vi "Write Read.vi"(8 "error in (no error)":errorcluster, 10 "Frames to Write":u16[](array[numeric]), 11 "SPI Ref In":T1={"myRIO Reference"={"myRIO Model"=enum."Unknown", "myRIO Hardware Reference"={"Generic FPGA Reference"=refnum, "Allow multiple opens"=FALSE}}, "SPI Channels Enum"=enum."Not Connected", "SPI Configuration"={"Frequency [Hz]"=0.0, "Clock Phase"=enum."Leading", "Clock Polarity"=enum."Low", "Data Direction"=enum."Most significant bit first", "Frame Length"=8}} {"SPI Configuration"."Frame Length" min=1 max=16}) -> (0 "error out":errorcluster, 2 "Frames Read":u16[](array[numeric]), 3 "SPI Ref Out":T1={"myRIO Reference"={"myRIO Model"=enum."Unknown", "myRIO Hardware Reference"={"Generic FPGA Reference"=refnum, "Allow multiple opens"=FALSE}}, "SPI Channels Enum"=enum."Not Connected", "SPI Configuration"={"Frequency [Hz]"=0.0, "Clock Phase"=enum."Leading", "Clock Polarity"=enum."Low", "Data Direction"=enum."Most significant bit first", "Frame Length"=8}} {"SPI Configuration"."Frame Length" min=1 max=16})   [LabVIEW 2021, in "SPI.lvlib"]
doc: "Writes and reads data frames through a serial peripheral interface (SPI) channel at the same time. The number of data frames to write equals the number of the data frames to read."
uses:
  <vilib>/myRIO/Instrument Drivers/Onboard IO/SPI/SPI.lvlib
  <vilib>/myRIO/Instrument Drivers/Onboard IO/SPI/typedefs/SPI Reference.ctl
  <vilib>/myRIO/Common/Instrument Driver Framework/Utilities/typedefs/myRIO Generic Hardware Reference.ctl
  <vilib>/myRIO/Common/Instrument Driver Framework/Utilities/typedefs/Hardware Version Enum.ctl
  <vilib>/myRIO/Common/Instrument Driver Framework/Utilities/typedefs/myRIO v1.0 Reference.ctl
  <vilib>/myRIO/Common/Instrument Driver Framework/Utilities/typedefs/Generic FPGA Reference.ctl
  <vilib>/myRIO/Common/Instrument Driver Framework/myRIO v1.0/SPI/typedefs/SPI Channels Enum.ctl
  <vilib>/myRIO/Instrument Drivers/Onboard IO/SPI/typedefs/SPI Configuration.ctl
  <vilib>/myRIO/Common/Instrument Driver Framework/myRIO v1.0/SPI/typedefs/SPI Clock Phase.ctl
  <vilib>/myRIO/Common/Instrument Driver Framework/myRIO v1.0/SPI/typedefs/SPI Clock Polarity.ctl
  <vilib>/myRIO/Common/Instrument Driver Framework/myRIO v1.0/SPI/typedefs/SPI Data Direction.ctl
  <vilib>/myRIO/Common/Instrument Driver Framework/myRIO v1.0/SPI/typedefs/SPI Frame Length.ctl
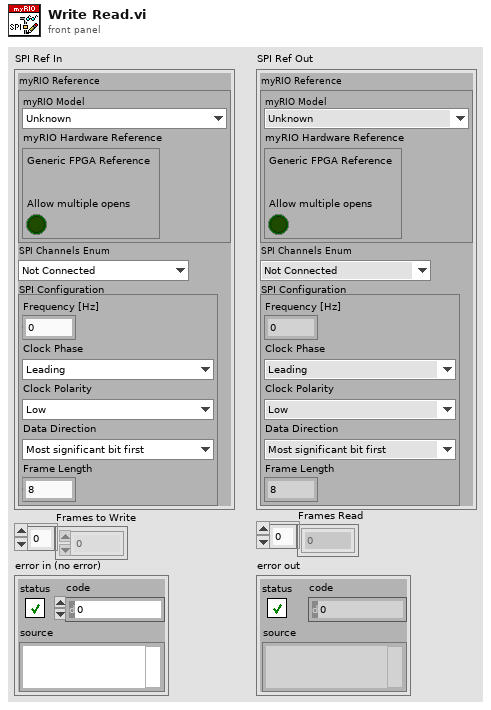
[diagram p1: front panel]
types:
  T1 = typedef "SPI.lvlib/SPI Reference.ctl" = cluster{"myRIO Reference":T2, "SPI Channels Enum":T6, "SPI Configuration":T7}
  T2 = typedef "myRIO Generic Hardware Reference.ctl" = cluster{"myRIO Model":T3, "myRIO Hardware Reference":T4}
  T3 = typedef "Hardware Version Enum.ctl" = enum16{"Unknown", "myRIO-1900", "myRIO-1950", "roboRIO", "NI ELVIS RIO CM", "ELVIS III"}
  T4 = typedef "myRIO v1.0 Reference.ctl" = cluster{"Generic FPGA Reference":T5, "Allow multiple opens":bool}
  T5 = typedef "Generic FPGA Reference.ctl" = refnum<k20>
  T6 = typedef "SPI Channels Enum.ctl" = enum16{"Not Connected", "A/SPI", "B/SPI", "SPI/SPI"}
  T7 = typedef "SPI.lvlib/SPI Configuration.ctl" = cluster{"Frequency [Hz]":dbl, "Clock Phase":T8, "Clock Polarity":T9, "Data Direction":T10, "Frame Length":T11}
  T8 = typedef "SPI Clock Phase.ctl" = enum8{"Leading", "Trailing"}
  T9 = typedef "SPI Clock Polarity.ctl" = enum8{"Low", "High"}
  T10 = typedef "SPI Data Direction.ctl" = enum8{"Most significant bit first", "Least significant bit first"}
  T11 = typedef "SPI Frame Length.ctl" = u8
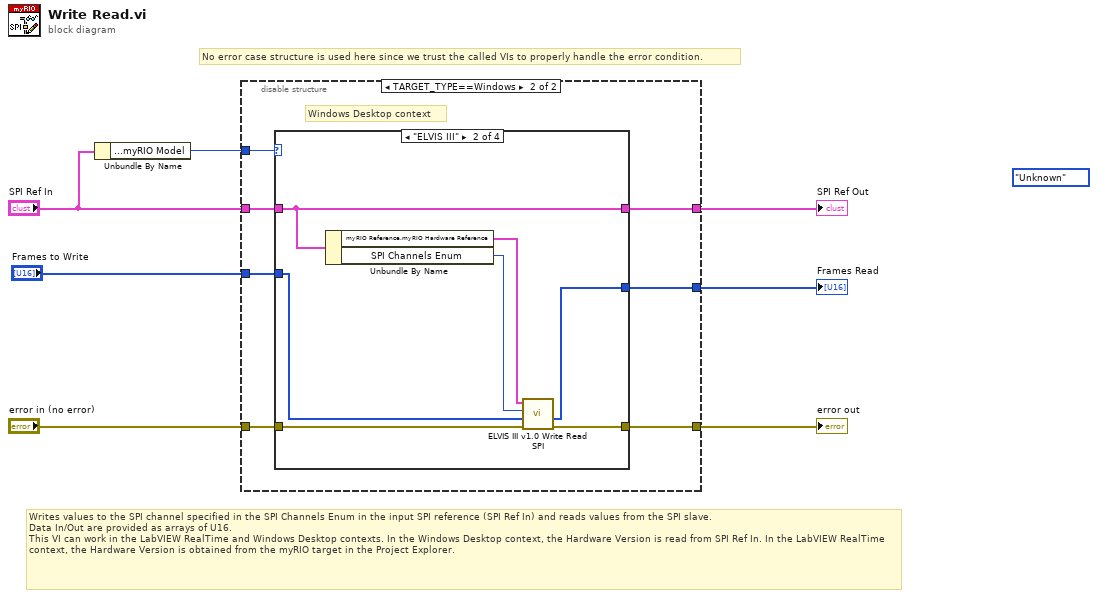
[diagram p0: block diagram]
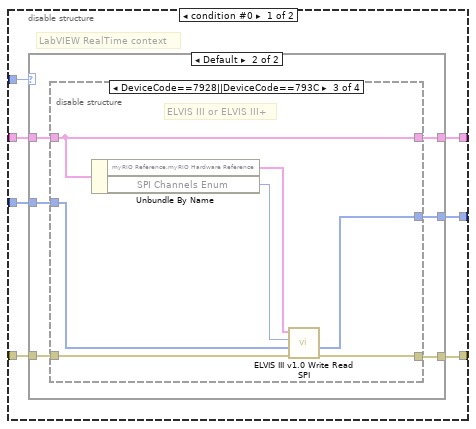
[diagram p2: hidden frame]
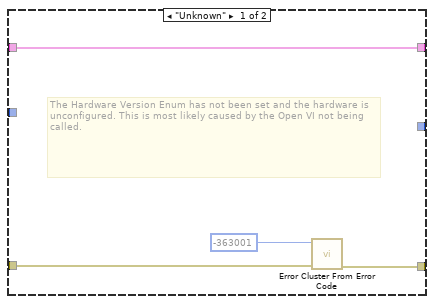
[diagram p3: hidden frame]
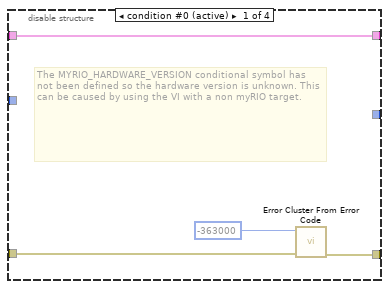
[diagram p4: hidden frame]
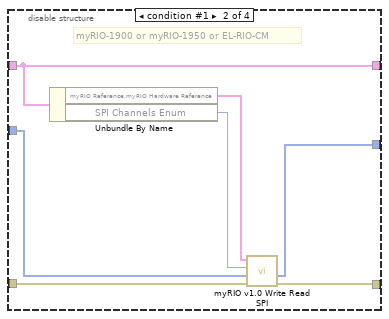
[diagram p5: hidden frame]
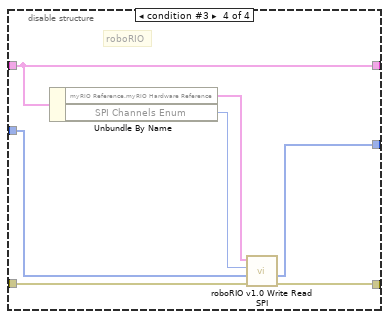
[diagram p6: hidden frame]
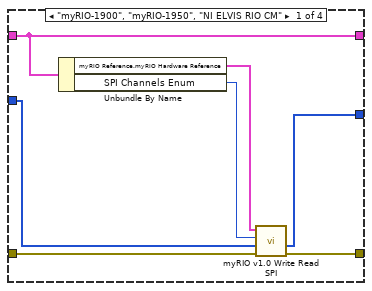
[diagram p7: hidden frame]
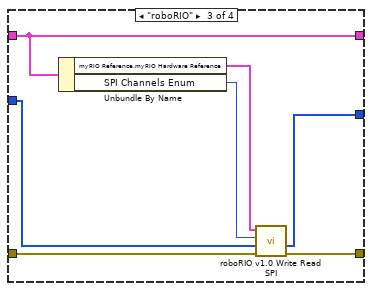
[diagram p8: hidden frame]
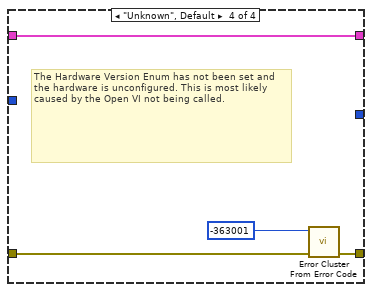
[diagram p9: hidden frame]
diagram:
  (unwired) Hardware_Version_Enum."Unknown" ("myRIO Reference.myRIO Model")
  # "No error case structure is used here since we trust the called VIs to properly handle the error condition."
  # "Writes values to the SPI channel specified in the SPI Channels Enum in the input SPI reference (SPI Ref In) and reads values from the SPI slave.\nData In/Out are provided as arrays of U16.\nThis VI can work in the LabVIEW RealTime and Windows Desktop contexts. In the Windows Desktop context, the Hardware Version is read from SPI Ref In. In the LabVIEW RealTime context, the Hardware Version is obtained from the myRIO target in the Project Explorer."
  n1 = Unbundle By Name("SPI Ref In") -> ("myRIO Reference.myRIO Model"=w1:T3)
  n2 = disable-structure shown="TARGET_TYPE==Windows" {
    disable-tunnel: [w14 w56] -> w4
    disable-tunnel: "SPI Ref In" -> [w13 w53]
    disable-tunnel: "error in (no error)" -> [w12 w55]
    disable-tunnel: [w11 w54] -> w5
    disable-tunnel: w1 -> [w10 w52]
    disable-tunnel: "Frames to Write" -> [w9 w51]
    disable-tunnel: [w8 w50] -> w2
    frame condition #0 {
      # "LabVIEW RealTime context"
      n3 = case shown="Default" w10 {
        tunnel: [w17 w24] -> w14
        tunnel: w13 -> [w15 w23]
        tunnel: w12 -> [w16 w22]
        tunnel: [w15 w21] -> w11
        tunnel: w9 -> [_ w20]
        tunnel: [_ w19] -> w8
        frame "Unknown" {
          # "The Hardware Version Enum has not been set and the hardware is unconfigured. This is most likely caused by the Open VI not being called."
          n4 = call <vilib>:"Error Cluster From Error Code.vi"("error in (no error)"=w16, "error code (0)"=-363001) -> ("error out"=w17:errorcluster)  [unwired: 7 in]
        }
        frame Default {
          n5 = disable-structure shown="DeviceCode==7928||DeviceCode==793C" {
            disable-tunnel: w23 -> [w25 w33 w40 w47]
            disable-tunnel: [w28 w31 w37 w45] -> w24
            disable-tunnel: w22 -> [w26 w32 w38 w46]
            disable-tunnel: [w25 w33 w40 w47] -> w21
            disable-tunnel: w20 -> [_ w30 w39 w44]
            disable-tunnel: [_ w29 w36 w43] -> w19
            frame condition #0 (active) {
              # "The MYRIO_HARDWARE_VERSION conditional symbol has not been defined so the hardware version is unknown. This can be caused by using the VI with a non myRIO target."
              n6 = call <vilib>:"Error Cluster From Error Code.vi"("error in (no error)"=w26, "error code (0)"=-363000) -> ("error out"=w28:errorcluster)  [unwired: 7 in]
            }
            frame condition #1 {
              # "myRIO-1900 or myRIO-1950 or EL-RIO-CM"
              n7 = Unbundle By Name(w33) -> ("myRIO Reference.myRIO Hardware Reference"=w35:T4, "SPI Channels Enum"=w34:T6)
              n8 = call <vilib>:"myRIO v1.0 Write Read SPI.vi"("error in (no error)"=w32, "Data In"=w30, "Channel"=w34, "myRIO Ref In"=w35) -> ("error out"=w31:errorcluster, "Data Out"=w29:u16[])  [unwired: 5 in, 1 out]
            }
            frame condition #2 {
              # "ELVIS III or ELVIS III+"
              n9 = Unbundle By Name(w40) -> ("myRIO Reference.myRIO Hardware Reference"=w42:T4, "SPI Channels Enum"=w41:T6)
              n10 = call <vilib>:"ELVIS III v1.0 Write Read SPI.vi"("error in (no error)"=w38, "Data In"=w39, "Channel"=w41, "myRIO Ref In"=w42) -> ("error out"=w37:errorcluster, "Data Out"=w36:u16[])  [unwired: 5 in, 1 out]
            }
            frame condition #3 {
              # "roboRIO"
              n11 = Unbundle By Name(w47) -> ("myRIO Reference.myRIO Hardware Reference"=w49:T4, "SPI Channels Enum"=w48:T6)
              n12 = call <vilib>:"roboRIO v1.0 Write Read SPI.vi"("error in (no error)"=w46, "Data In"=w44, "Channel"=w48, "myRIO Ref In"=w49) -> ("error out"=w45:errorcluster, "Data Out"=w43:u16[])  [unwired: 5 in, 1 out]
            }
          }
        }
      }
    }
    frame condition #1 (active) {
      # "Windows Desktop context"
      n13 = case shown="\"ELVIS III\"" w52 {
        tunnel: [w60 w66 w74 w81] -> w56
        tunnel: w53 -> [w61 w68 w75 w78]
        tunnel: w55 -> [w59 w64 w73 w79]
        tunnel: [w61 w68 w75 w78] -> w54
        tunnel: w51 -> [w58 w65 w72 _]
        tunnel: [w57 w67 w71 _] -> w50
        frame "myRIO-1900", "myRIO-1950", "NI ELVIS RIO CM" {
          n14 = Unbundle By Name(w61) -> ("myRIO Reference.myRIO Hardware Reference"=w63:T4, "SPI Channels Enum"=w62:T6)
          n15 = call <vilib>:"myRIO v1.0 Write Read SPI.vi"("error in (no error)"=w59, "Data In"=w58, "Channel"=w62, "myRIO Ref In"=w63) -> ("error out"=w60:errorcluster, "Data Out"=w57:u16[])  [unwired: 5 in, 1 out]
        }
        frame "ELVIS III" {
          n16 = Unbundle By Name(w68) -> ("myRIO Reference.myRIO Hardware Reference"=w70:T4, "SPI Channels Enum"=w69:T6)
          n17 = call <vilib>:"ELVIS III v1.0 Write Read SPI.vi"("error in (no error)"=w64, "Data In"=w65, "Channel"=w69, "myRIO Ref In"=w70) -> ("error out"=w66:errorcluster, "Data Out"=w67:u16[])  [unwired: 5 in, 1 out]
        }
        frame "roboRIO" {
          n18 = Unbundle By Name(w75) -> ("myRIO Reference.myRIO Hardware Reference"=w77:T4, "SPI Channels Enum"=w76:T6)
          n19 = call <vilib>:"roboRIO v1.0 Write Read SPI.vi"("error in (no error)"=w73, "Data In"=w72, "Channel"=w76, "myRIO Ref In"=w77) -> ("error out"=w74:errorcluster, "Data Out"=w71:u16[])  [unwired: 5 in, 1 out]
        }
        frame "Unknown", Default {
          # "The Hardware Version Enum has not been set and the hardware is unconfigured. This is most likely caused by the Open VI not being called."
          n20 = call <vilib>:"Error Cluster From Error Code.vi"("error in (no error)"=w79, "error code (0)"=-363001) -> ("error out"=w81:errorcluster)  [unwired: 7 in]
        }
      }
    }
  }
  "SPI Ref Out" <- w5
  "error out" <- w4
  "Frames Read" <- w2
